vi "PicoScope5000aOpen.vi"(0 "USB 3.0 device on non-USB 3.0 Port control":bool=TRUE, 7 "Serial Number":string, 8 "USB Powered control":bool=TRUE, 9 "Resolution":i32(ring) items=["8-bit", "12-bit", "14-bit", "15-bit (max. 2 ch.)", "16-bit (max. 1 ch.)"], 10 "Use Serial Number":bool, 11 "error in (no error)":errorcluster) -> (1 "USB Powered":bool=TRUE, 2 "handle":i16, 3 "error out":errorcluster, 4 "Max ADC value":i16, 5 "USB 3.0 device on non-USB 3.0 Port":bool=TRUE, 6 "Device Info":T1)   [LabVIEW 2020]
doc: "This VI opens a PicoScope 3000a/b and returns a handle to the device."
uses:
  ps5000a.dll
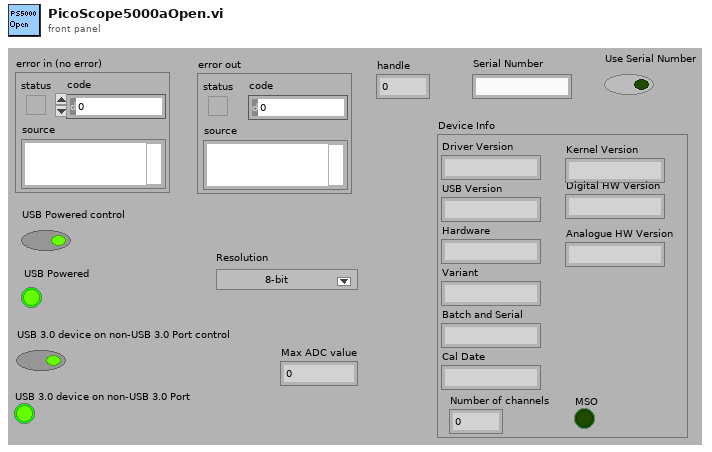
[diagram p1: front panel]
types:
  T1 = cluster{"Driver Version":string, "USB Version":string, "Hardware":string, "Variant":string, "Batch and Serial":string, "Cal Date":string, "Kernel Version":string, "Digital HW Version":string, "Analogue HW Version":string, "MSO":bool, "Number of channels":i16}
  T2 = cluster{"Driver Version":string, "USB Version":string, "Hardware":string, "Variant":string, "Batch and Serial":string, "Cal Date":string, "Kernel Version":string, "Digital HW Version":string, "Analogue HW Version":string, "Firmware 1":string, "Firmware 2":string}
  T3 = cluster{"Driver Version":string, "USB Version":string, "Hardware":string, "Variant":string, "Batch and Serial":string, "Cal Date":string, "Kernel Version":string, "Digital HW Version":string, "Analogue HW Version":string, bool, i16}
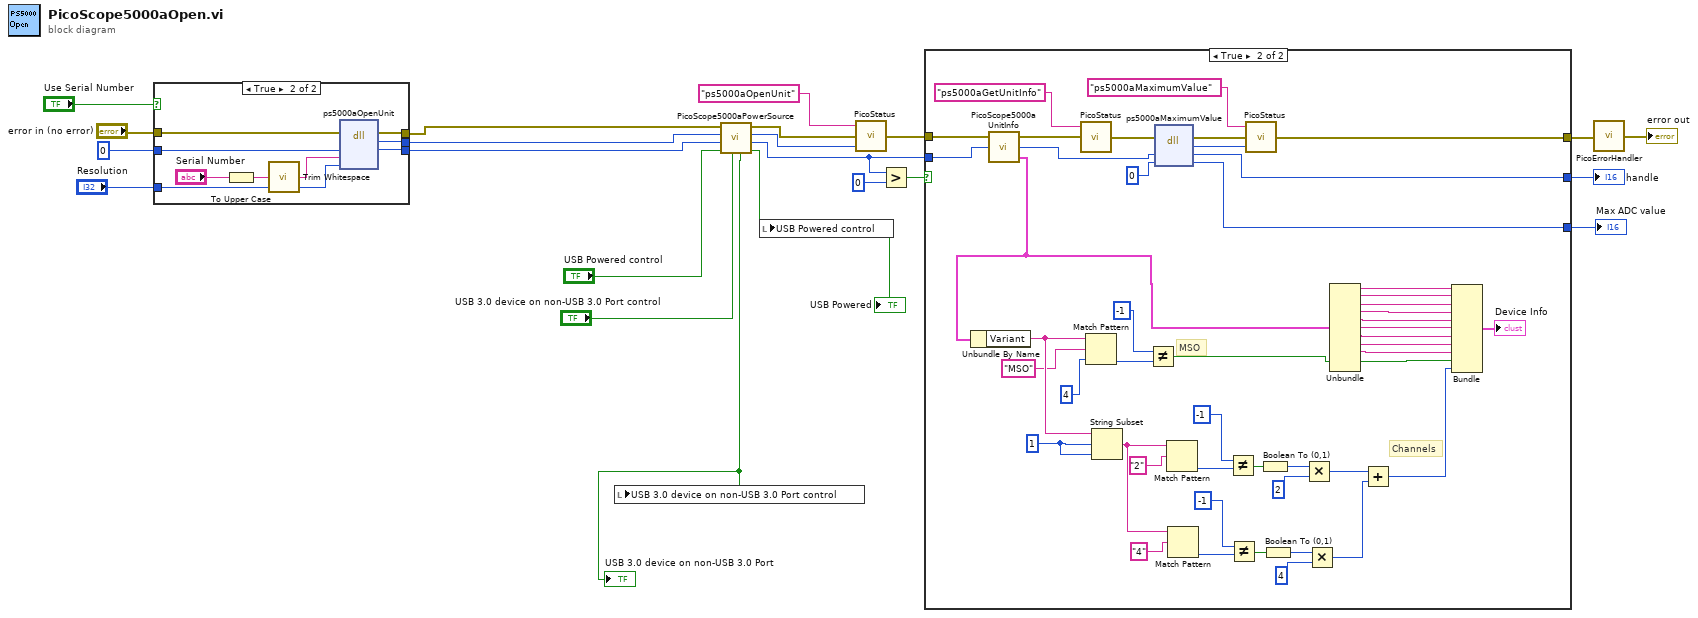
[diagram p0: block diagram]
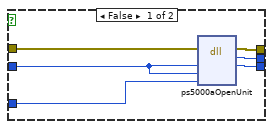
[diagram p2: hidden frame]
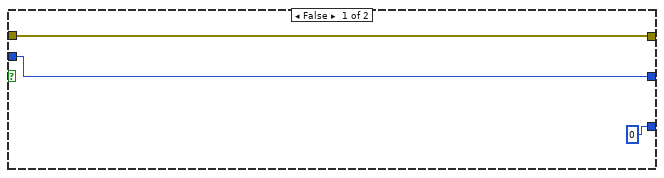
[diagram p3: hidden frame]
diagram:
  n1 = case shown="True" "Use Serial Number" {
    tunnel: "error in (no error)" -> [w28 w33]
    tunnel: i16 0 ("handle") -> [w23 w34]
    tunnel: [w27 w37] -> w18
    tunnel: [w26 w36] -> w16
    tunnel: [w25 w35] -> w15
    tunnel: "Resolution" -> [w24 w32]
    frame False {
      n2 = dll-call lib="ps5000a.dll" fn="ps5000aOpenUnit" ("ps3000.dll:_ps3000_open_unit@0")(error in=w28, "handle"=w23, "serial"=w23, "resolution"=w24) -> (error out=w27:errorcluster, "PICO_STATUS"=w26:i32, "handle"=w25:i16)  [unwired: 4 in, 1 out]
    }
    frame True {
      n3 = To Upper Case(1:"Serial Number") -> (0:w30:string)
      n4 = call "Trim Whitespace.vi"("string"=w30) -> ("trimmed string"=w29:string)  [unwired: 1 in]
      n5 = dll-call lib="ps5000a.dll" fn="ps5000aOpenUnit" ("ps3000.dll:_ps3000_open_unit@0")(error in=w33, "handle"=w34, "serial"=w29, "resolution"=w32) -> (error out=w37:errorcluster, "PICO_STATUS"=w36:u32, "handle"=w35:i16)  [unwired: 4 in, 1 out]
    }
  }
  n6 = call "PicoScope5000aPowerSource.vi"("USB 3.0 on non-USB 3.0 port control"="USB 3.0 device on non-USB 3.0 Port control", "USB Powered control"="USB Powered control", "handle in"=w15, "PICO STATUS IN"=w16, "error in (no error)"=w18) -> ("USB Powered"=w12:bool, "handle out"=w7:i16, "PICO STATUS OUT"=w14:u32, "error out"=w17:errorcluster, "USB 3.0 on non-USB 3.0 Port"=w1:bool)  [unwired: 2 in]
  "USB Powered" <- w12
  "USB 3.0 device on non-USB 3.0 Port" <- w1
  n7 = local write "USB 3.0 device on non-USB 3.0 Port control"(w1) -> ()
  n8 = local write "USB Powered control"(w12) -> ()
  n9 = call "PicoStatus.vi"("PICO STATUS"=w14, "error in"=w17, "source"="ps5000aOpenUnit") -> ("error out"=w11:errorcluster)
  n10 = Greater?(x=w7, y=0) -> (0:w8:bool)
  n11 = case shown="True" w8 {
    tunnel: w7 -> [w39 w87]
    tunnel: w11 -> [w40 w86]
    tunnel: [w40 w46] -> w10
    tunnel: [w39 w44] -> w9
    tunnel: [i16 0 ("value") w42] -> w3
    frame False {
    }
    frame True {
      w74 = 1 ("offset (0)")
      # "MSO"
      # "Channels"
      n12 = call "PicoScope5000aUnitInfo.vi"("handle in"=w87, "error in (no error)"=w86) -> ("Unit Info"=w50:T2, "handle out"=w48:i16, "error out"=w85:errorcluster)  [unwired: 1 in]
      n13 = Unbundle By Name(w50) -> ("Variant"=w70:string)
      n14 = call "PicoStatus.vi"("error in"=w85, "source"="ps5000aGetUnitInfo") -> ("error out"=w49:errorcluster)  [unwired: 1 in]
      n15 = Match Pattern(string=w70, regular expression="MSO", offset (0)=4) -> (offset past match=w67:i32)  [unwired: 3 out]
      n16 = String Subset(string=w70, offset (0)=w74, length (rest)=w74) -> (substring=w61:string)
      n17 = Not Equal?(x=-1, y=w67) -> (x != y?=w65:bool)
      n18 = dll-call lib="ps5000a.dll" fn="ps5000aMaximumValue"(error in=w49, "handle"=w48, "value"=i16 0) -> (error out=w47:errorcluster, "PICO_STATUS"=w45:u32, "handle"=w44:i16, "value"=w42:i16)  [unwired: 2 in, 1 out]
      n19 = Match Pattern(string=w61, regular expression="2") -> (offset past match=w72:i32)  [unwired: 1 in, 3 out]
      n20 = Match Pattern(string=w61, regular expression="4") -> (offset past match=w63:i32)  [unwired: 1 in, 3 out]
      n21 = Not Equal?(x=-1, y=w72) -> (x != y?=w57:bool)
      n22 = Not Equal?(x=-1, y=w63) -> (x != y?=w53:bool)
      n23 = call "PicoStatus.vi"("PICO STATUS"=w45, "error in"=w47, "source"="ps5000aMaximumValue") -> ("error out"=w46:errorcluster)
      n24 = Boolean To (0,1)(Boolean=w57) -> (0, 1=w56:i16)
      n25 = Boolean To (0,1)(Boolean=w53) -> (0, 1=w54:i16)
      n26 = Multiply(x=w56, y=i16 2) -> (x*y=w60:i16)
      n27 = Multiply(x=w54, y=i16 4) -> (x*y=w52:i16)
      n28 = Unbundle(w50) -> ("Driver Version"=w83:string, "USB Version"=w82:string, "Hardware"=w81:string, "Variant"=w80:string, "Batch and Serial"=w79:string, "Cal Date"=w78:string, "Kernel Version"=w77:string, "Digital HW Version"=w76:string, "Analogue HW Version"=w75:string)  [unwired: 2 out]
      n29 = Add(x=w60, y=w52) -> (x+y=w59:i16)
      n30 = Bundle("Driver Version"=w83, "USB Version"=w82, "Hardware"=w81, "Variant"=w80, "Batch and Serial"=w79, "Cal Date"=w78, "Kernel Version"=w77, "Digital HW Version"=w76, "Analogue HW Version"=w75, w65, w59) -> (→"Device Info":T3)  [unwired: 1 in]
    }
  }
  "handle" <- w9
  "Max ADC value" <- w3
  n31 = call "PicoErrorHandler.vi"("error in"=w10) -> ("error out"=→"error out":errorcluster)
